vi "Cieślikiewicz1_2.vi"() -> ()   [LabVIEW 2020]
panel:
  out "Waveform Chart":dbl[](graph)
  in  "stop":bool
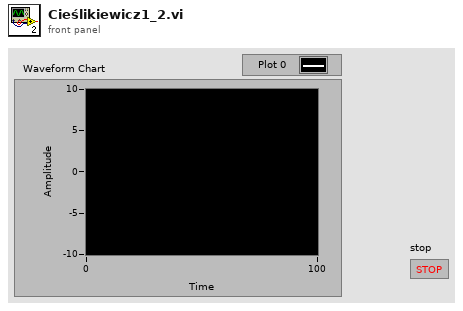
[diagram p1: front panel]
types:
  T1 = typedef "Rendezvous RefNum" = refnum<k1>
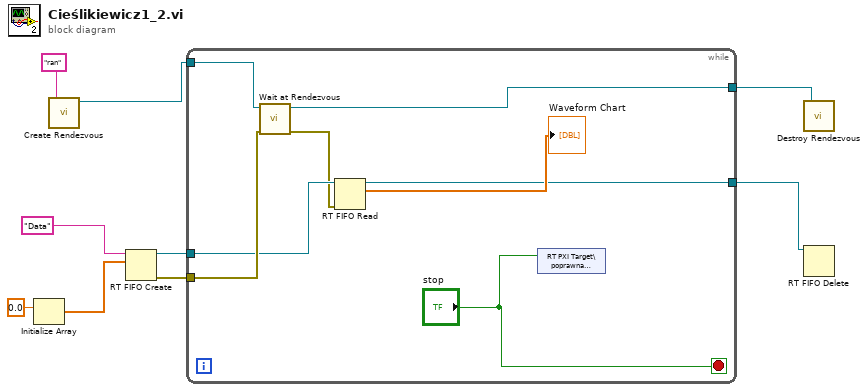
[diagram p0: block diagram]
diagram:
  n1 = Initialize Array(0.0 ("element")) -> (w8:dbl[])  [unwired: 1 in]
  n2 = call <vilib>:"Create Rendezvous.vi"("name (unnamed)"="ran") -> ("rendezvous"=w1:T1)  [unwired: 4 in, 2 out]
  n3 = RT FIFO Create(0:"Data" ("name (unnamed)"), 1:w8) -> (8:w6:refnum<k33>, 11:w5:errorcluster)  [unwired: 6 in, 1 out]
  n4 = while {
    tunnel: w6 -> [w16]
    tunnel: w5 -> [w17]
    tunnel: [w14] -> w4
    tunnel: [w13] -> w3
    tunnel: w1 -> [w12]
    stop <- "stop" stop-if-true
    n5 = call <vilib>:"Wait at Rendezvous.vi"("error in (no error)"=w17, "rendezvous"=w12) -> ("error out"=w11:errorcluster, "rendezvous out"=w13:T1)  [unwired: 3 in, 1 out]
    n6 = RT FIFO Read(0:w16, 3:w11) -> (8:w14:refnum<k33>, 9:→"Waveform Chart":dbl[])  [unwired: 2 in, 3 out]
    n7 = shared-variable "RT PXI Target\\poprawna bilbioteka.lvlib\\stop"("stop") -> ()  [unwired: 1 in, 1 out]
  }
  n8 = call <vilib>:"Destroy Rendezvous.vi"("rendezvous"=w3) -> ()  [unwired: 5 in, 2 out]
  n9 = RT FIFO Delete(0:w4) -> ()  [unwired: 2 in, 1 out]
